vi "From hab right to far rocket.vi"   [LabVIEW 2018]
uses:
  Drive/Implementation/Drive Operations.ctl
  Path Data.ctl
  Framework/Robot Global Data.vi
types:
  T1 = typedef "Path Data.ctl" = cluster{"Maneuver":enum16{"MAX 90", "MAX 180", "Turn to Home", "Turn to Rocket", "Auto-Align"}, "Rotation Direction":enum16{"N/A", "Right", "Left"}}[]
  T2 = typedef "Drive Operations.ctl" = enum16{"Reserve", "Read Current", "Immediate", "J-Turn", "Play Back From Log", "Auto-Align"}
  T3 = typedef "Command Status Info.ctl" = cluster{"Name":string, "Status":T4, "notifier out":T5}
  T4 = typedef "Completion Status.ctl" = enum16{"Successful", "Aborted", "Incomplete"}
  T5 = typedef "Completion Notifier.ctl" = refnum<notifier>
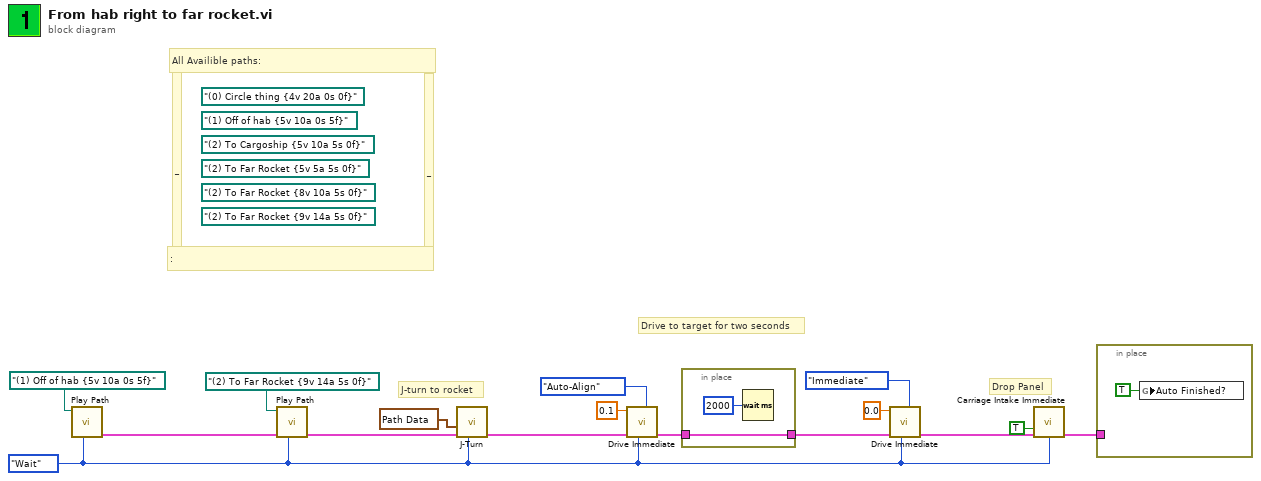
[diagram p0: block diagram]
diagram:
  (unwired) path "(2) To Far Rocket {5v 5a 5s 0f}"
  (unwired) path "(2) To Far Rocket {8v 10a 5s 0f}"
  (unwired) path "(2) To Cargoship {5v 10a 5s 0f}"
  (unwired) path "(2) To Far Rocket {9v 14a 5s 0f}"
  (unwired) path "(1) Off of hab {5v 10a 0s 5f}"
  w6 = enum16{"Start", "Wait"}."Wait" ("Synchronication")
  (unwired) path "(0) Circle thing {4v 20a 0s 0f}"
  # "Drop Panel"
  # "Drive to target for two seconds"
  # ":"
  # "_"
  # "_"
  # "All Availible paths:"
  # "J-turn to rocket"
  n1 = call "Play Path.vi"("Synchronication"=w6, "Path"=path "(1) Off of hab {5v 10a 0s 5f}") -> ("Command Info Out"=w14:T3)  [unwired: 9 in]
  n2 = call "Play Path.vi"("Synchronication"=w6, "Command Info In"=w14, "Path"=path "(2) To Far Rocket {9v 14a 5s 0f}") -> ("Command Info Out"=w1:T3)  [unwired: 8 in]
  n3 = call "J-Turn.vi"("Synchronication"=w6, "Command Info In"=w1, "Path Data"=T1 [{"Maneuver"=enum."Auto-Align", "Rotation Direction"=enum."N/A"}, {"Maneuver"=enum."MAX 90", "Rotation Direction"=enum."N/A"}, {"Maneuver"=enum."MAX 90", "Rotation Direction"=enum."N/A"}]) -> ("Command Info Out"=w12:T3)  [unwired: 8 in]
  n4 = call "Drive Immediate.vi"("Operation"=Drive_Operations."Auto-Align", "Synchronication"=w6, "Command Info In"=w12, "Left Setpoint (Power)"=0.1) -> ("Command Info Out"=w9:T3)  [unwired: 7 in]
  n5 = in-place {
    in-place-border: w9 -> [w18]
    in-place-border: [w18] -> w8
    n6 = Wait (ms)(milliseconds to wait=u32 2000) -> ()  [unwired: 1 out]
  }
  n7 = call "Drive Immediate.vi"("Operation"=Drive_Operations."Immediate", "Synchronication"=w6, "Command Info In"=w8, "Left Setpoint (Power)"=0.0) -> ("Command Info Out"=w7:T3)  [unwired: 7 in]
  n8 = call "Carriage Intake Immediate.vi"("Close"=TRUE, "Command Info In"=w7, "Synchronication"=w6) -> ("Command Info Out"=w16:T3)  [unwired: 12 in]
  n9 = in-place {
    in-place-border: w16 -> [_]
    n10 = global write "Robot Global Data.vi" "Auto Finished?"(TRUE ("Auto Finished?")) -> ()
  }
